vi "__Init Front Panel Controls.vi"(8 "error in (no error)":errorcluster, 11 "FileManager Ctl Refs in":T1) -> (0 "error out":errorcluster, 3 "FileManager Ctl Refs out":T1)   [LabVIEW 2011]
doc: "Initializes all the front panel objects to their default value.\nThen refreshes the local and cloud lists."
uses:
  __File manager Data type.ctl
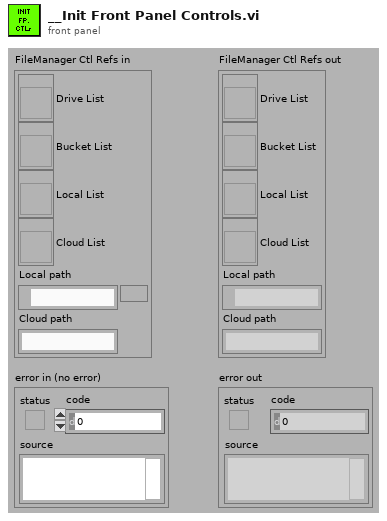
[diagram p1: front panel]
types:
  T1 = typedef "__File manager Data type.ctl" = cluster{"Drive List":refnum<vi>, "Bucket List":refnum<vi>, "Local List":refnum<vi>, "Cloud List":refnum<vi>, "Local path":path, "Cloud path":string}
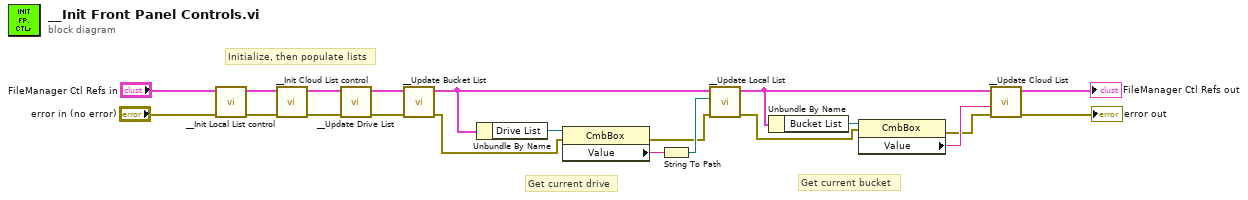
[diagram p0: block diagram]
diagram:
  # "Get current bucket"
  # "Get current drive"
  # "Initialize, then populate lists"
  n1 = call "__Init Local List control.vi"("error in (no error)"="error in (no error)", "FileManager Ctl Refs in"="FileManager Ctl Refs in") -> ("error out"=w19:errorcluster, "FileManager Ctl Refs out"=w20:T1)  [unwired: 8 in]
  n2 = call "__Init Cloud List control.vi"("error in (no error)"=w19, "FileManager Ctl Refs in"=w20) -> ("error out"=w18:errorcluster, "FileManager Ctl Refs out"=w17:T1)  [unwired: 8 in]
  n3 = call "__Update Drive List.vi"("error in (no error)"=w18, "FileManager Ctl Refs in"=w17) -> ("error out"=w16:errorcluster, "FileManager Ctl Refs out"=w15:T1)  [unwired: 8 in]
  n4 = call "__Update Bucket List.vi"("error in (no error)"=w16, "FileManager Ctl Refs in"=w15) -> ("error out"=w13:errorcluster, "FileManager Ctl Refs out"=w10:T1)  [unwired: 8 in]
  n5 = Unbundle By Name(w10) -> ("Drive List"=w14:refnum<vi>)
  n6 = property class="CmbBox"(reference=w14, error in=w13) -> (error out=w9:errorcluster, "Value"=w12:string)  [unwired: 1 out]
  n7 = String To Path(string=w12) -> (path=w11:path)
  n8 = call "__Update Local List.vi"("error in (no error)"=w9, "Path to list"=w11, "FileManager Ctl Refs in"=w10) -> ("error out"=w6:errorcluster, "FileManager Ctl Refs out"=w7:T1)  [unwired: 7 in]
  n9 = Unbundle By Name(w7) -> ("Bucket List"=w8:refnum<vi>)
  n10 = property class="CmbBox"(reference=w8, error in=w6) -> (error out=w4:errorcluster, "Value"=w5:string)  [unwired: 1 out]
  n11 = call "__Update Cloud List.vi"("error in (no error)"=w4, "Bucket"=w5, "FileManager Ctl Refs in"=w7) -> ("error out"=→"error out":errorcluster, "FileManager Ctl Refs out"=→"FileManager Ctl Refs out":T1)  [unwired: 7 in]
